vi "Save Preset SubVI.vi"(6 "Preset Save":bool, 7 "Control Settings":refnum<vi>[](array[refnum]), 8 "error in (no error)":errorcluster, 9 "Preset Directory:":path, 11 "Preset Name":string) -> (0 "error out":errorcluster, 2 "Reset 'Preset Save'":bool=TRUE)   [LabVIEW 2018]
uses:
  Load and Save Controls_LV2009.llb/RWC_Actions.ctl
  <vilib>/Utility/config.llb/NI_LVConfig.lvlib
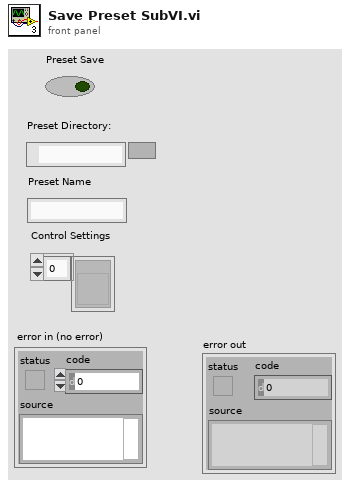
[diagram p1: front panel]
types:
  T1 = typedef "RWC_Actions.ctl" = enum16{"Read", "Write", "Read and Create"}
  T2 = typedef "NI_LVConfig.lvlib/Config Data RefNum.ctl" = refnum<k1>
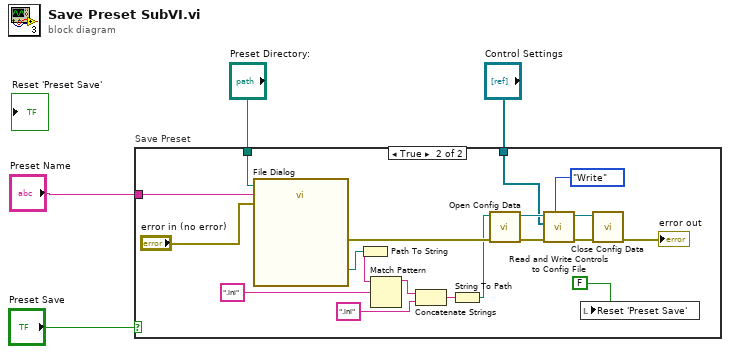
[diagram p0: block diagram]
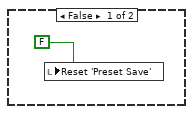
[diagram p2: hidden frame]
diagram:
  n1 = case "Save Preset" shown="True" "Preset Save" {
    tunnel: "Control Settings" -> [_ w21]
    tunnel: "Preset Directory:" -> [_ w20]
    tunnel: "Preset Name" -> [_ w7]
    frame False {
      n2 = local write "Reset 'Preset Save'"(FALSE ("Start Custom Test")) -> ()
    }
    frame True {
      n3 = call "File Dialog"("start path"=w20, "default name"=w7, "error in"="error in (no error)") -> ("selected path"=w14:path, "error out"=w19:errorcluster)  [unwired: 9 in, 2 out]
      n4 = Path To String(path=w14) -> (string=w9:string)
      n5 = Match Pattern(string=w9, regular expression=".ini") -> (before substring=w8:string)  [unwired: 1 in, 3 out]
      n6 = Concatenate Strings(w8, ".ini") -> (w13:string)
      n7 = String To Path(string=w13) -> (path=w11:path)
      n8 = call <vilib>:"Open Config Data.vi"("error in (no error)"=w19, "configuration file path"=w11) -> ("error out"=w18:errorcluster, "refnum"=w23:T2)  [unwired: 7 in, 1 out]
      n9 = call "Read and Write Controls to Config File.vi"("Action"=RWC_Actions."Write", "error in"=w18, "Control References"=w21, "Configuration File Reference In"=w23) -> ("error out"=w17:errorcluster, "Configuration File Reference Out"=w24:T2)  [unwired: 6 in]
      n10 = local write "Reset 'Preset Save'"(FALSE ("Start Custom Test")) -> ()
      n11 = call <vilib>:"Close Config Data.vi"("error in (no error)"=w17, "refnum"=w24) -> ("error out"=→"error out":errorcluster)  [unwired: 8 in, 1 out]
    }
  }
